vi "GSP_filtererrorcode.vi"(0 "error in (no error)":errorcluster, 1 "Filter Codes":i32[](array[numeric])) -> (5 "filtered error":errorcluster)   [LabVIEW 2015]
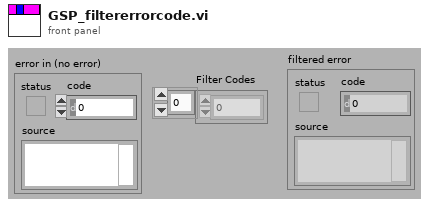
[diagram p1: front panel]
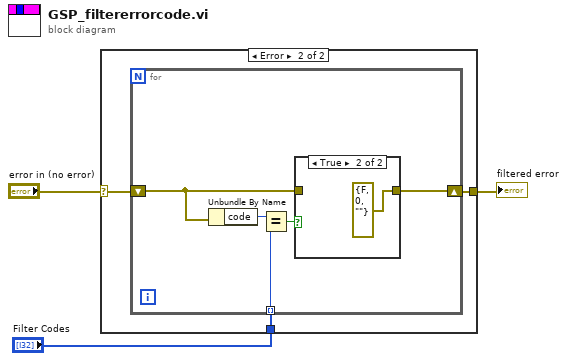
[diagram p0: block diagram]
diagram:
  n1 = case shown="Error" "error in (no error)" {
    selector: "error in (no error)" -> [w4 w5]
    tunnel: "Filter Codes" -> [_ w7]
    tunnel: [w4 w6] -> w2
    frame No Error {
    }
    frame Error {
      n2 = for {
        tunnel: w7 -> [w12] mode=indexing
        shift-right: [w10] -> w6
        shift-left: w5 -> [w11]
        n3 = Unbundle By Name(w11) -> ("code"=w9:i32)
        n4 = Equal?(x=w9, y=w12) -> (x = y?=w8:bool)
        n5 = case shown="True" w8 {
          tunnel: w11 -> [w13 _]
          tunnel: [w13 errorcluster {"status"=FALSE, "code"=0, "source"=""} ("error IO")] -> w10
          frame False {
          }
          frame True {
          }
        }
      }
    }
  }
  "filtered error" <- w2
